vi "ELVIS III v1.0 Reserve UART.vi"(8 "error in (no error)":errorcluster, 10 "VISA resource name in":refnum<visa-resource-name>, 11 "myRIO FPGA Ref In":T1) -> (0 "error out":errorcluster)   [LabVIEW 2021]
uses:
  <vilib>/myRIO/Common/Instrument Driver Framework/Utilities/typedefs/Generic FPGA Reference.ctl
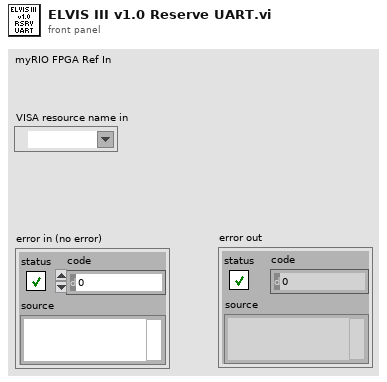
[diagram p1: front panel]
types:
  T1 = typedef "Generic FPGA Reference.ctl" = refnum<k20>
  T2 = typedef "ELVIS III v1.0 Channel Reservation List.ctl" = T3[]
  T3 = typedef "ELVIS III v1.0 Channel Reservation Info.ctl" = cluster{"Channel Name":string, "Connector":T4, "MutexIDs":u32[]}
  T4 = typedef "ELVIS III v1.0 Connector List.ctl" = enum32{"None", "ConnectorA", "ConnectorB"}
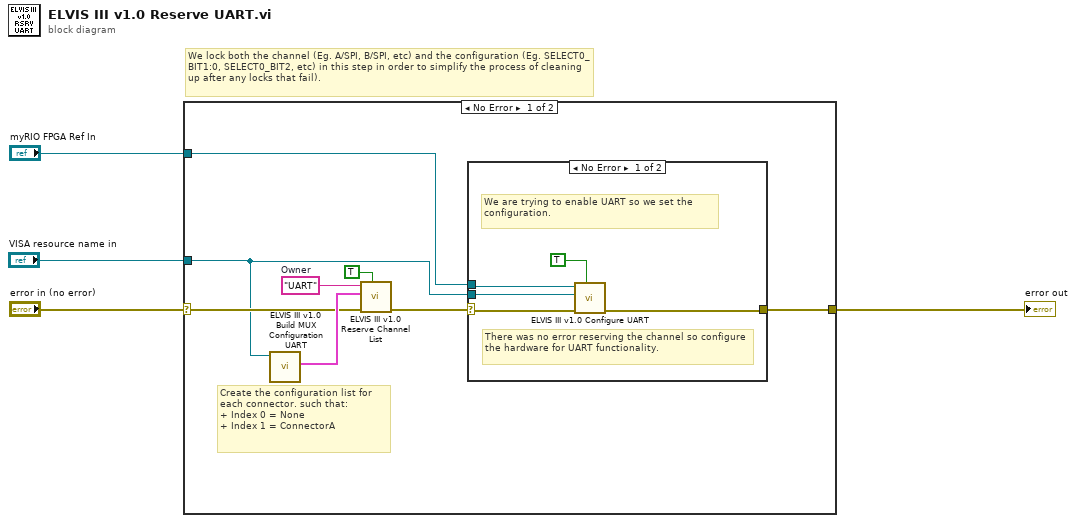
[diagram p0: block diagram]
diagram:
  # "We lock both the channel (Eg. A/SPI, B/SPI, etc) and the configuration (Eg. SELECT0_BIT1:0, SELECT0_BIT2, etc) in this step in order to simplify the process of cleaning up after any locks that fail)."
  n1 = case shown="No Error" "error in (no error)" {
    selector: "error in (no error)" -> [w8 w19]
    tunnel: "myRIO FPGA Ref In" -> [w11 _]
    tunnel: "VISA resource name in" -> [w6 _]
    tunnel: [w10 w19] -> w3
    frame No Error {
      w12 = "UART"  # Owner
      # "Create the configuration list for each connector. such that:\n+ Index 0 = None\n+ Index 1 = ConnectorA"
      n2 = call <vilib>:"ELVIS III v1.0 Build MUX Configuration UART.vi"("VISA resource name in"=w6) -> ("Channel Reservation List"=w9:T2)  [unwired: 10 in]
      n3 = call <vilib>:"ELVIS III v1.0 Reserve Channel List.vi"("Allow multiple opens?"=TRUE, "error in (no error)"=w8, "Channel Reservation List"=w9, "Owner"=w12) -> ("error out"=w7:errorcluster)  [unwired: 7 in]
      n4 = case shown="No Error" w7 {
        selector: w7 -> [w17 w18]
        tunnel: w11 -> [w14 _]
        tunnel: [w16 w18] -> w10
        tunnel: w6 -> [w15 _]
        frame No Error {
          # "There was no error reserving the channel so configure the hardware for UART functionality."
          # "We are trying to enable UART so we set the configuration."
          n5 = call <vilib>:"ELVIS III v1.0 Configure UART.vi"("Reserve?"=TRUE, "error in (no error)"=w17, "VISA resource name in"=w15, "myRIO FPGA Ref"=w14) -> ("error out"=w16:errorcluster)  [unwired: 7 in]
        }
        frame Error {
        }
      }
    }
    frame Error {
      # "Nothing to do since there is an incoming error."
    }
  }
  "error out" <- w3
